vi "SetVIDescription&Help.vi"(4 "Help Tag":string, 6 "Help Path":string, 9 "VI Description":string, 10 "VI Index":i32, 11 "VI Data in":T1[](array[typedef])) -> (3 "VI Data out":T1[](array[typedef]))   [LabVIEW 2016, in "update vi properties.lvlib"]
uses:
  update vi properties.lvlib
  Cluster_Data.ctl
  <vilib>/picture/picture.llb/imagedata.ctl
panel:
  # "Connector Pane"
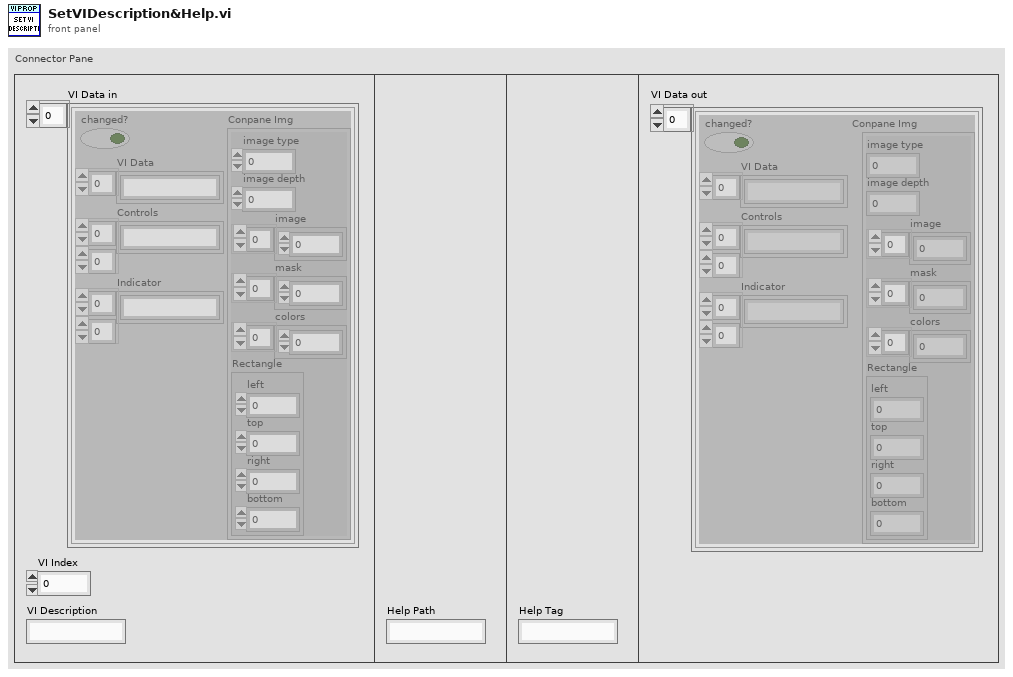
[diagram p1: front panel]
types:
  T1 = typedef "update vi properties.lvlib/Cluster_Data.ctl" = cluster{"changed?":bool, "VI Data":string[], "Controls":string[][], "Indicator":string[][], "Conpane Img":T2}
  T2 = typedef "imagedata.ctl" = cluster{"image type":i32, "image depth":i32, "image":u8[], "mask":u8[], "colors":u32[], "Rectangle":cluster{"left":i16, "top":i16, "right":i16, "bottom":i16}}
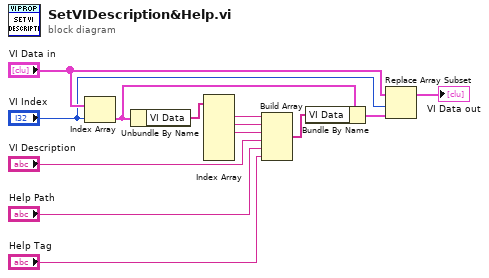
[diagram p0: block diagram]
diagram:
  n1 = Index Array(array="VI Data in", index="VI Index") -> (element=w3:T1)
  n2 = Unbundle By Name(w3) -> ("VI Data"=w13:string[])
  n3 = Index Array(array=w13) -> (element #1=w5:string, element #2=w4:string, element #3=w6:string)  [unwired: 6 in, 3 out]
  n4 = Build Array(w5, w4, w6, "VI Description", "Help Path", "Help Tag") -> (w2:string[])
  n5 = Bundle By Name(cluster=w3, "VI Data"=w2) -> (w1:T1)
  n6 = Replace Array Subset(array="VI Data in", new element=w1, index="VI Index") -> (→"VI Data out":T1[])
